vi "RBF Weights.vi"(9 "RBF Weights in":dbl[](array[numeric]), 11 "RBF Weights before":dbl[](array[numeric])) -> (2 "RBF Weights out":dbl[](array[numeric]), 3 "RBF Weights before":dbl[](array[numeric]))   [LabVIEW 2021]
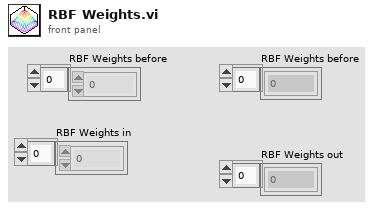
[diagram p1: front panel]
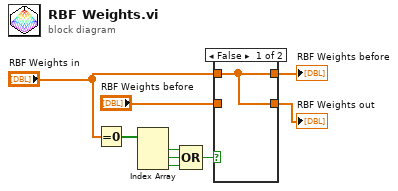
[diagram p0: block diagram]
diagram:
  n1 = Equal To 0?(x="RBF Weights in") -> (x = 0?=w9:bool[])
  n2 = Index Array(array=w9) -> (element #1=w7:bool, element #2=w3:bool, element #3=w2:bool)  [unwired: 3 in]
  n3 = Compound Arithmetic op=OR(w7, w3, w2) -> (w8:bool)
  n4 = case shown="False" w8 {
    tunnel: [w10 w11] -> w4
    tunnel: "RBF Weights before" -> [_ w11]
    tunnel: [w10 w11] -> w6
    tunnel: "RBF Weights in" -> [w10 _]
    frame False {
    }
    frame True {
    }
  }
  "RBF Weights out" <- w6
  "RBF Weights before" <- w4
